vi "Initialize Generate.vi"(8 "error in (no error)":errorcluster, 10 "Target Ref in":T8 format="%.0x", 11 "Addon Ref in":T8 format="%.0x") -> (0 "error out":errorcluster, 2 "Found?":bool, 3 "Generate Frame Configurations":T1[](array[typedef]) {"CD Results Refs"."Data Reference" format="%.0x"; "Input Channels Refs"."Data Reference" format="%.0x"; "Frame Configuration"."CRCConfiguration"."FinalXorValue" format="%0x"; "Frame Configuration"."CRCConfiguration"."InitialCRC" format="%0x"; "Frame Configuration"."CRCConfiguration"."Polynomial" format="%0x"; "Frame Configuration"."CRC"."Data Type" items=["Signed", "Unsigned", "IEEE Float"]; "Frame Configuration"."Rolling Counter"."Data Type" items=["Signed", "Unsigned", "IEEE Float"]; "Frame Configuration"."Input Channels"."Data Type" items=["Signed", "Unsigned", "IEEE Float"]})   [LabVIEW 2021, in "LIN Frame Protection Addon Engine.lvlib"]
uses:
  LIN Frame Protection Addon Engine.lvlib
  <vilib>/NI VeriStand/Custom Device API/Custom Device Item Ref.ctl
  Types/RT Engine Generate References.ctl
  Shared/Types/FrameConfiguration.ctl
  Shared/Types/InputChannelConfiguration.ctl
  Shared/Types/Protection Type.ctl
  Shared/Types/CRCConfiguration.ctl
  <vilib>/NI VeriStand/Custom Device API/Block Data Reference.ctl
  <vilib>/NI VeriStand/Custom Device API/Data Reference.ctl
  <vilib>/NI VeriStand/Custom Device Tools/Custom Device Utility Library/Search Direction.ctl
  <vilib>/NI VeriStand/Custom Device API/Data Access Type.ctl
  Shared/SubVIs/GUID Lookup.vi
  <vilib>/NI VeriStand/Custom Device Tools/Custom Device Utility Library/NI VeriStand - Search for Item by GUID.vi
  <vilib>/NI VeriStand/Custom Device Tools/Custom Device Utility Library/NI VeriStand - Search for All Items by GUID.vi
  <vilib>/xnet/xnet.llb/XNET Create Session (Conversion).vi
  <vilib>/NI VeriStand/Custom Device Tools/Custom Device Utility Library/Custom Device Utility Library.lvlib
  Shared/LIN Frame Protection Addon Shared.lvlib
  <vilib>/NI VeriStand/Custom Device API/Custom Device API.lvlib
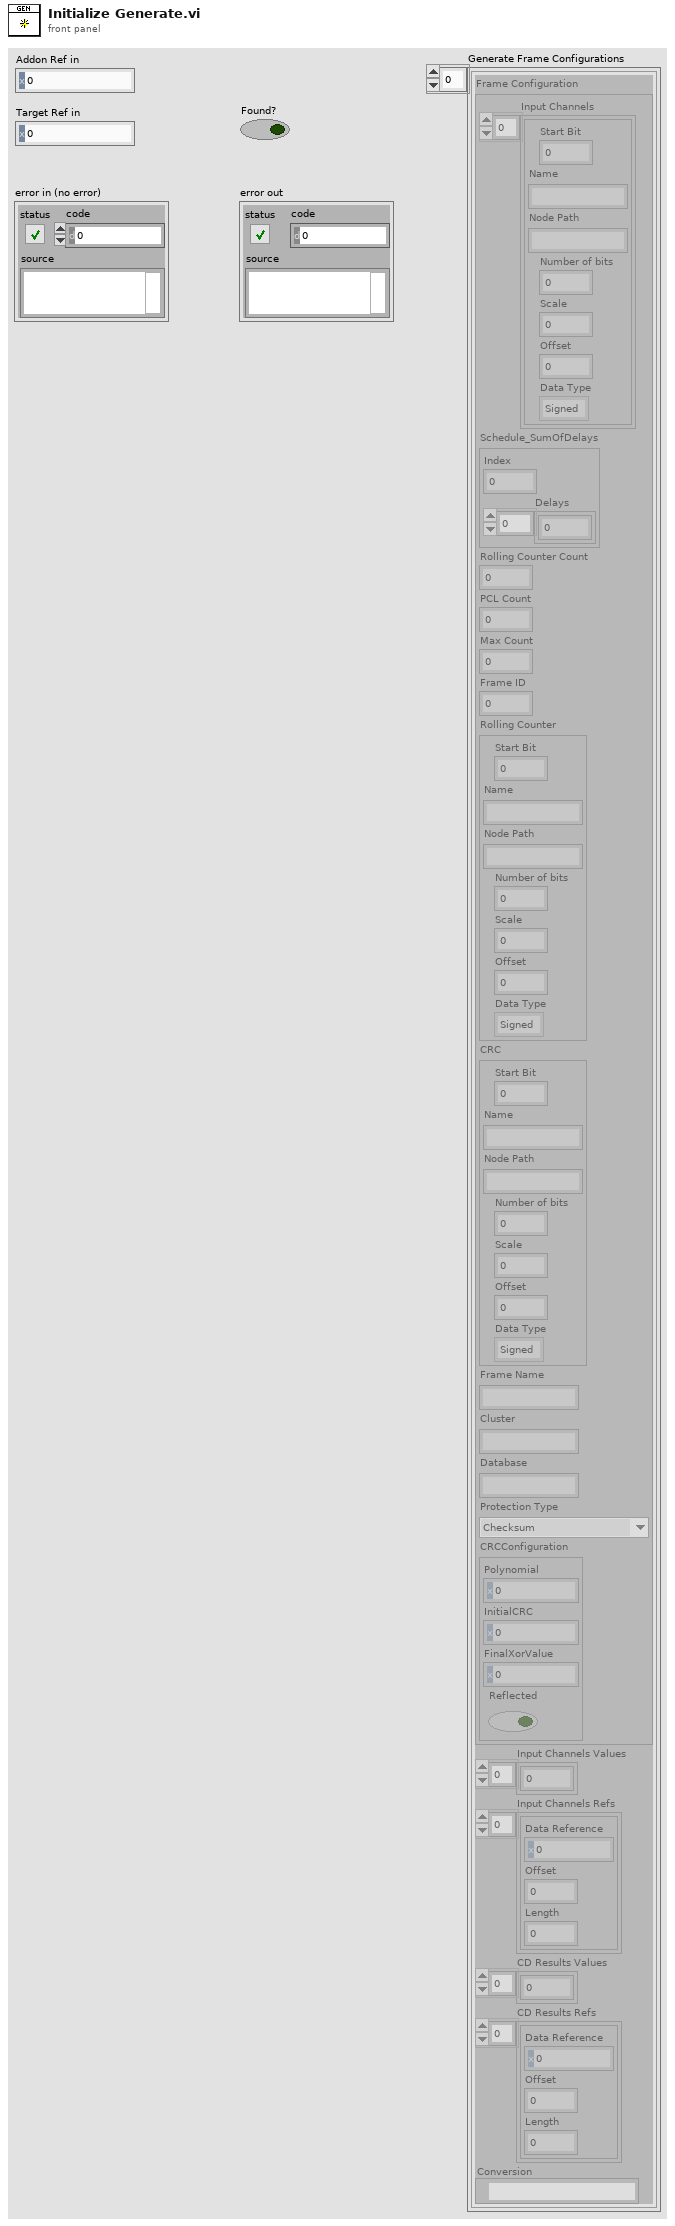
[diagram p1: front panel]
types:
  T1 = typedef "LIN Frame Protection Addon Engine.lvlib/RT Engine Generate References.ctl" = cluster{"Frame Configuration":T2, "Input Channels Values":dbl[], "Input Channels Refs":T6[], "CD Results Values":dbl[], "CD Results Refs":T6[], "Conversion":refnum<k21>}
  T2 = typedef "LIN Frame Protection Addon Shared.lvlib/FrameConfiguration.ctl" = cluster{"Input Channels":T3[], "Schedule_SumOfDelays":cluster{"Index":i32, "Delays":dbl[]}, "Rolling Counter Count":dbl, "PCL Count":u64, "Max Count":dbl, "Frame ID":u32, "Rolling Counter":T3, "CRC":T3, "Frame Name":string, "Cluster":string, "Database":string, "Protection Type":T4, "CRCConfiguration":T5}
  T3 = typedef "LIN Frame Protection Addon Shared.lvlib/InputChannelConfiguration.ctl" = cluster{"Start Bit":i32, "Name":string, "Node Path":string, "Number of bits":i32, "Scale":dbl, "Offset":dbl, "Data Type":u32}
  T4 = typedef "LIN Frame Protection Addon Shared.lvlib/Protection Type.ctl" = enum16{"Checksum", "CRC-8", "CRC-16", "CRC-32", "None (Counter Only)"}
  T5 = typedef "LIN Frame Protection Addon Shared.lvlib/CRCConfiguration.ctl" = cluster{"Polynomial":u64, "InitialCRC":u64, "FinalXorValue":u64, "Reflected":bool}
  T6 = typedef "Custom Device API.lvlib/Block Data Reference.ctl" = cluster{"Data Reference":T7, "Offset":u64, "Length":u64}
  T7 = typedef "Custom Device API.lvlib/Data Reference.ctl" = i32
  T8 = typedef "Custom Device API.lvlib/Custom Device Item Ref.ctl" = u64
  T9 = typedef "Custom Device Utility Library.lvlib/Search Direction.ctl" = enum16{"Down", "Up"}
  T10 = typedef "Custom Device API.lvlib/Data Access Type.ctl" = enum16{"Read", "Write"}
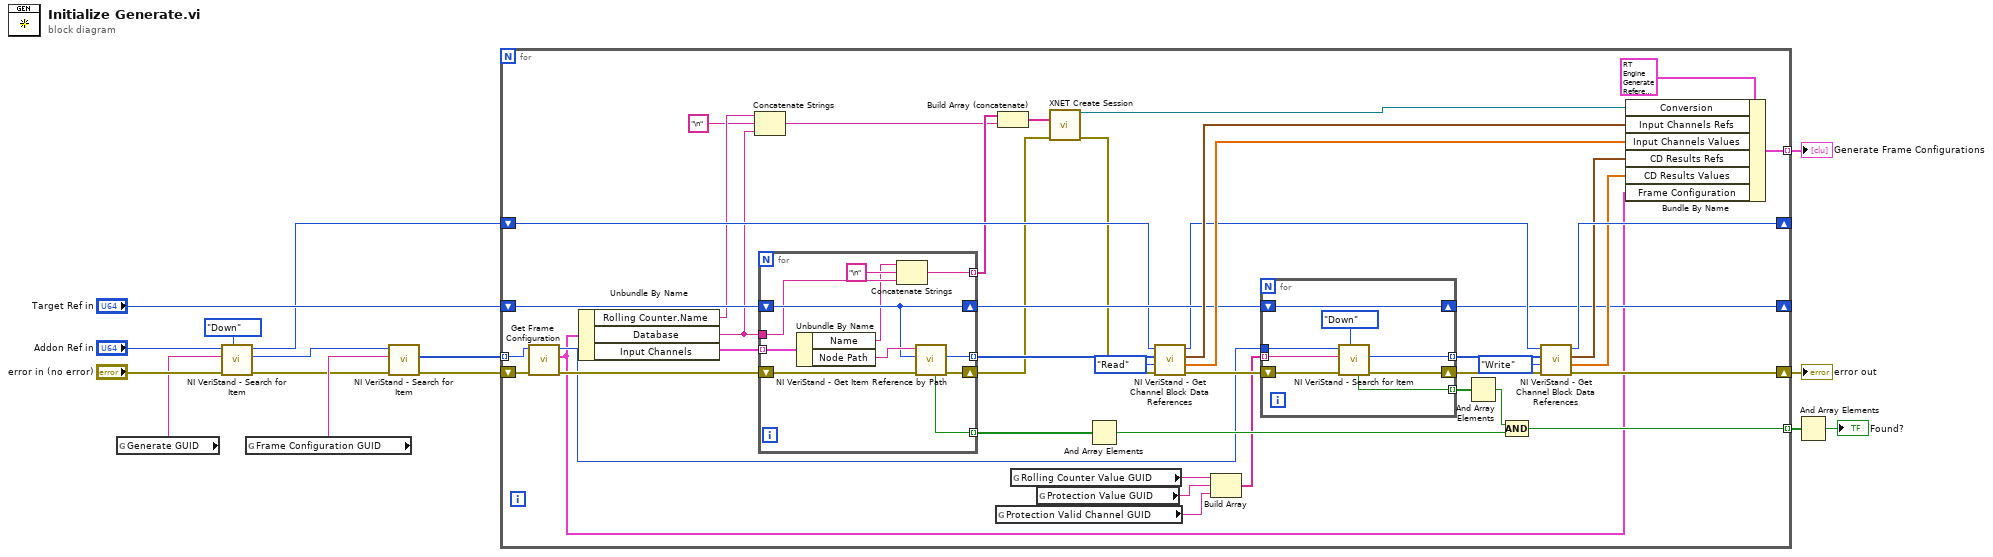
[diagram p0: block diagram]
diagram:
  n1 = global read "GUID Lookup.vi" "Generate GUID"() -> (w4:string)
  n2 = call-poly <vilib>:"NI VeriStand - Search for Item.vi"("Direction (Down)"=Search_Direction."Down", "error in"="error in (no error)", "Item GUID"=w4, "Section Ref in"="Addon Ref in") -> ("error out"=w8:errorcluster, "Item Ref"=w6:T8, "Section Ref out"=w5:T8)  [unwired: 4 in, 1 out]
  n3 = global read "GUID Lookup.vi" "Frame Configuration GUID"() -> (w10:string)
  n4 = call-poly <vilib>:"NI VeriStand - Search for Item.vi"("error in"=w8, "Item GUID"=w10, "Section Ref in"=w6) -> ("error out"=w11:errorcluster, "Item Refs"=w12:T8[])  [unwired: 5 in, 2 out]
  n5 = for {
    shift-right: [w37] -> w14
    shift-left: w11 -> [w58]
    tunnel: w12 -> [w57] mode=indexing
    shift-right: [w49] -> _
    shift-left: w5 -> [w32]
    tunnel: [w41] -> w2 mode=indexing
    tunnel: [w44] -> w13 mode=indexing
    shift-right: [w27] -> _
    shift-left: "Target Ref in" -> [w34]
    n6 = call "Get Frame Configuration.vi"("error in"=w58, "Parent Ref"=w57) -> ("error out"=w33:errorcluster, "Selected Channels"=w16:T2, "Parent Ref Out"=w31:T8)  [unwired: 7 in]
    n7 = Unbundle By Name(w16) -> ("Rolling Counter.Name"=w23:string, "Database"=w21:string, "Input Channels"=w56:T3[])
    n8 = Concatenate Strings(w23, "\n" ("string"), w21) -> (w20:string)
    n9 = for {
      tunnel: w56 -> [w77] mode=indexing
      shift-right: [w73] -> w18
      shift-left: w33 -> [w76]
      shift-right: [w71] -> w36
      shift-left: w34 -> [w71]
      tunnel: [w75] -> w52 mode=indexing
      tunnel: [w74] -> w55 mode=indexing
      tunnel: w21 -> [w69]
      tunnel: [w67] -> w25 mode=indexing
      n10 = Unbundle By Name(w77) -> ("Name"=w68:string, "Node Path"=w72:string)
      n11 = Concatenate Strings(w68, "\n" ("string"), w69) -> (w67:string)
      n12 = call <vilib>:"NI VeriStand - Get Item Reference by Path.vi"("error in (no error)"=w76, "Root Ref"=w71, "Item Path in"=w72) -> ("error out"=w73:errorcluster, "Item Ref"=w75:T8, "Found"=w74:bool)  [unwired: 5 in, 1 out]
    }
    n13 = global read "GUID Lookup.vi" "Protection Valid Channel GUID"() -> (w26:string)
    n14 = Build Array (concatenate)(w25, w20) -> (w24:string[])
    n15 = global read "GUID Lookup.vi" "Rolling Counter Value GUID"() -> (w30:string)
    n16 = global read "GUID Lookup.vi" "Protection Value GUID"() -> (w29:string)
    n17 = call-poly <vilib>:"XNET Create Session.vi"("signal list"=w24, "error in (no error)"=w18) -> ("session out"=w19:refnum<k21>, "error out"=w17:errorcluster)  [unwired: 12 out]
    n18 = And Array Elements(Boolean array=w55) -> (logical AND=w54:bool)
    n19 = call <vilib>:"NI VeriStand - Get Channel Block Data References.vi"("error in (no error)"=w17, "Access"=Data_Access_Type."Read", "Channel Refs"=w52, "Device Ref in"=w32) -> ("error out"=w39:errorcluster, "Values Array"=w50:dbl[], "Block Data Refs"=w51:T6[], "Device Ref out"=w35:T8)  [unwired: 4 in]
    n20 = Build Array(w30, w29, w26) -> (w28:string[])
    n21 = for {
      shift-right: [w64] -> w38
      shift-left: w39 -> [w65]
      shift-right: [w66] -> w27
      shift-left: w36 -> [w66]
      tunnel: [w62] -> w45 mode=indexing
      tunnel: [w63] -> w42 mode=indexing
      tunnel: w31 -> [w61]
      tunnel: w28 -> [w60] mode=indexing
      n22 = call-poly <vilib>:"NI VeriStand - Search for Item.vi"("Direction (Down)"=Search_Direction."Down", "error in"=w65, "Item GUID"=w60, "Section Ref in"=w61) -> ("error out"=w64:errorcluster, "Item Ref"=w62:T8, "Found"=w63:bool)  [unwired: 4 in, 1 out]
    }
    n23 = And Array Elements(Boolean array=w42) -> (logical AND=w40:bool)
    n24 = Compound Arithmetic op=AND(w40, w54) -> (w41:bool)
    n25 = call <vilib>:"NI VeriStand - Get Channel Block Data References.vi"("error in (no error)"=w38, "Access"=Data_Access_Type."Write", "Channel Refs"=w45, "Device Ref in"=w35) -> ("error out"=w37:errorcluster, "Values Array"=w46:dbl[], "Block Data Refs"=w47:T6[], "Device Ref out"=w49:T8)  [unwired: 4 in]
    n26 = Bundle By Name(cluster=T1 {"Frame Configuration"={"Input Channels"=[], "Schedule_SumOfDelays"={"Index"=0, "Delays"=[]}, "Rolling Counter Count"=0.0, "PCL Count"=0, "Max Count"=0.0, "Frame ID"=0, "Rolling Counter"={"Start Bit"=0, "Name"="", "Node Path"="", "Number of bits"=0, "Scale"=0.0, "Offset"=0.0, "Data Type"=0}, "CRC"={"Start Bit"=0, "Name"="", "Node Path"="", "Number of bits"=0, "Scale"=0.0, "Offset"=0.0, "Data Type"=0}, "Frame Name"="", "Cluster"="", "Database"="", "Protection Type"=enum."Checksum", "CRCConfiguration"={"Polynomial"=0, "InitialCRC"=0, "FinalXorValue"=0, "Reflected"=FALSE}}, "Input Channels Values"=[], "Input Channels Refs"=[], "CD Results Values"=[], "CD Results Refs"=[], "Conversion"=""} ("output cluster"), "Conversion"=w19, "Input Channels Refs"=w51, "Input Channels Values"=w50, "CD Results Refs"=w47, "CD Results Values"=w46, "Frame Configuration"=w16) -> (w44:T1)
  }
  "error out" <- w14
  "Generate Frame Configurations" <- w13
  n27 = And Array Elements(Boolean array=w2) -> (logical AND=→"Found?":bool)
